vi "4.5.vi"() -> ()   [LabVIEW 2017]
panel:
  out "随机数":dbl
  out "循环次数":i32
  in  "指定值":dbl
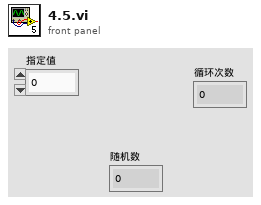
[diagram p1: front panel]
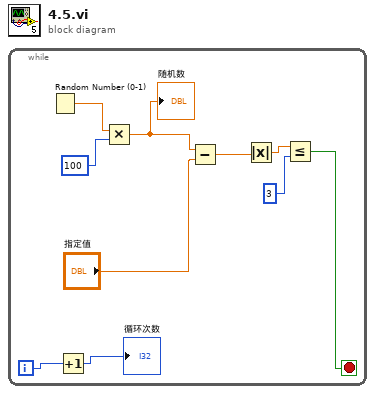
[diagram p0: block diagram]
diagram:
  n1 = while {
    i -> [w3]
    stop <- w4 stop-if-true
    n2 = Random Number (0-1)() -> (number: 0 to 1=w10:dbl)
    n3 = Increment(x=w3) -> (x+1=→"循环次数":i32)
    n4 = Multiply(x=w10, y=100) -> (x*y=w1:dbl)
    "随机数" <- w1
    n5 = Subtract(x=w1, y="指定值") -> (x-y=w7:dbl)
    n6 = Absolute Value(x=w7) -> (abs(x)=w6:dbl)
    n7 = Less Or Equal?(x=w6, y=3) -> (x <= y?=w4:bool)
  }
